vi "Execute.vi"(0 "object in":refnum<class "Logger.lvclass">, 2 "Requirements":T2={"From"=enum."TDMS", "File Handler"=variant, "Input"=variant(map{string, dbl[]} {})}, 5 "Error In":errorcluster) -> (14 "object out":refnum<class "Logger.lvclass">, 16 "Message":T1, 19 "Error Out":errorcluster)   [LabVIEW 2024, in "Logger.lvclass"]
doc: "Logs given input data to target (From) file type"
uses:
  Logger.lvclass
  Support/Type Def/Requirements.ctl
  Support/Type Def/File Type.ctl
  Support/Type Def/Message.ctl
  Support/Type Def/Data.ctl
  <vilib>/Utility/file.llb/Write Delimited Spreadsheet (DBL).vi
panel:
  # "Connector Pane"
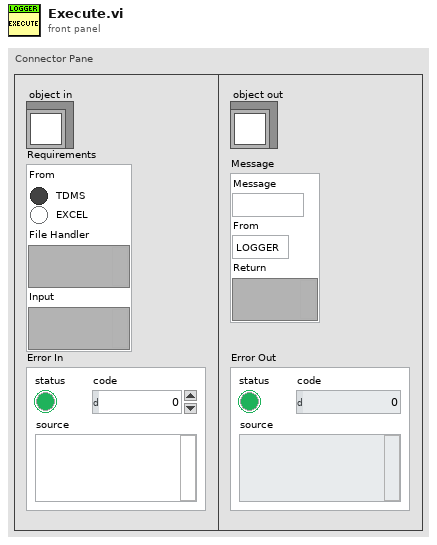
[diagram p1: front panel]
types:
  T1 = typedef "Message.ctl" = cluster{"Message":string, "From":enum16{"LOGGER", "VIEWER"}, "Return":variant}
  T2 = typedef "Requirements.ctl" = cluster{"From":T3, "File Handler":variant, "Input":variant}
  T3 = typedef "File Type.ctl" = enum32{"TDMS", "EXCEL"}
  T4 = typedef "Data.ctl" = map{string, dbl[]}
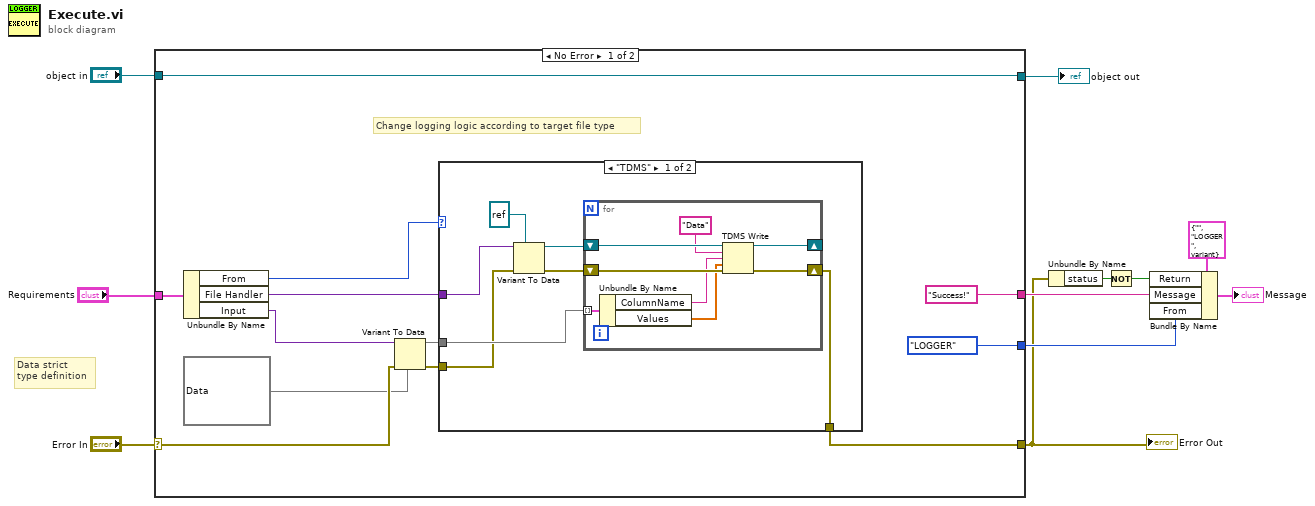
[diagram p0: block diagram]
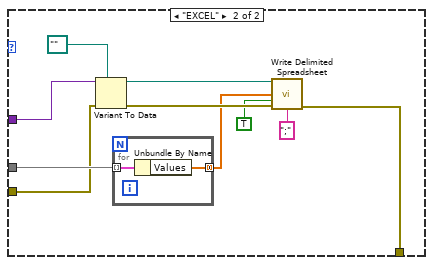
[diagram p2: hidden frame]
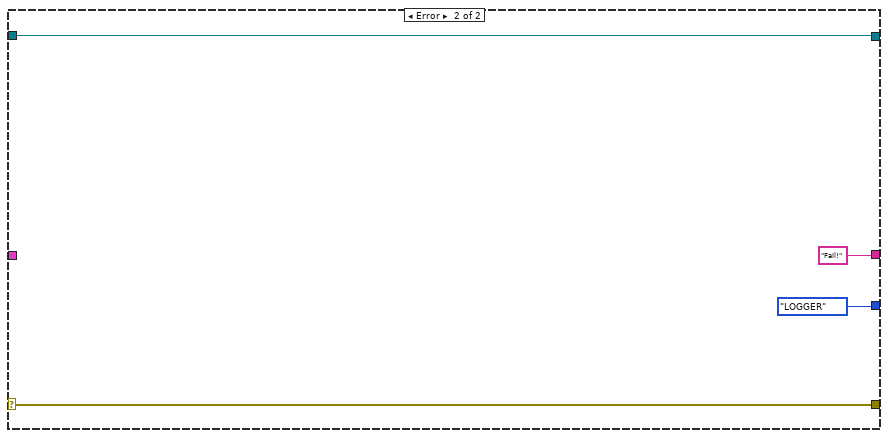
[diagram p3: hidden frame]
diagram:
  # "Data strict\ntype definition"
  n1 = case shown="No Error" "Error In" {
    selector: "Error In" -> [w13 w54]
    tunnel: [w18 w54] -> w3
    tunnel: [w23 w53] -> w9
    tunnel: "object in" -> [w23 w53]
    tunnel: "Requirements" -> [w22 _]
    tunnel: ["Success!" ("Message") "Fail!" ("Message")] -> w5
    tunnel: [enum16{"LOGGER", "VIEWER"}."LOGGER" ("From") enum16{"LOGGER", "VIEWER"}."LOGGER" ("From")] -> w4
    frame No Error {
      # "Change logging logic according to target file type"
      n2 = Unbundle By Name(w22) -> ("From"=w21:T3, "File Handler"=w20:variant, "Input"=w19:variant)
      n3 = Variant To Data(error in=w13, type=T4 {} ("Data"), Variant=w19) -> (data=w15:T4, error out=w14:errorcluster)
      n4 = case shown="\"TDMS\"" w21 {
        tunnel: w20 -> [w30 w48]
        tunnel: w15 -> [w28 w44]
        tunnel: [w26 w43] -> w18
        tunnel: w14 -> [w25 w42]
        frame "TDMS" {
          n5 = Variant To Data(error in=w25, type=refnum<k34> refnum ("tdms file"), Variant=w30) -> (data=w27:refnum<k34>, error out=w29:errorcluster)
          n6 = for {
            shift-right: [w35] -> _
            shift-left: w27 -> [w32]
            shift-right: [w36] -> w26
            shift-left: w29 -> [w37]
            tunnel: w28 -> [w38] mode=indexing
            n7 = Unbundle By Name(w38) -> ("ColumnName"=w33:string, "Values"=w34:dbl[])
            n8 = TDMS Write(0:w32, 5:"Data" ("group name in (Untitled)"), 7:w33, 9:w34, 11:w37) -> (4:w35:refnum<k34>, 15:w36:errorcluster)  [unwired: 1 in, 2 out]
          }
        }
        frame "EXCEL" {
          n9 = Variant To Data(error in=w42, type=path "" ("file path (dialog if empty)"), Variant=w48) -> (data=w46:path, error out=w45:errorcluster)
          n10 = for {
            tunnel: w44 -> [w50] mode=indexing
            tunnel: [w49] -> w39 mode=concatenating
            n11 = Unbundle By Name(w50) -> ("Values"=w49:dbl[])
          }
          n12 = call-poly <vilib>:"Write Delimited Spreadsheet.vi"("file path (dialog if empty)"=w46, "1D data"=w39, "append to file? (new file:F)"=TRUE, "error in (no error)"=w45, "delimiter (\\t)"=";" ("delimiter (\\t)")) -> ("error out"=w43:errorcluster)  [unwired: 9 in, 1 out]
        }
      }
    }
    frame Error {
    }
  }
  "Error Out" <- w3
  "object out" <- w9
  n13 = Unbundle By Name(w3) -> ("status"=w2:bool)
  n14 = Not(x=w2) -> (.not. x?=w1:bool)
  n15 = Bundle By Name(cluster=T1 {"Message"="", "From"=enum."LOGGER", "Return"=variant} ("Message"), "Return"=w1, "Message"=w5, "From"=w4) -> (→"Message":T1)
